vi "Write Caller Enqueuer.vi"(8 "error in (no error)":errorcluster, 10 "Actor Framework:Message Enqueuer":refnum<class "Message Enqueuer.lvclass">, 11 "Async Message in":refnum<class "Async Message.lvclass">) -> (0 "error out":errorcluster, 3 "Async Message out":refnum<class "Async Message.lvclass">)   [LabVIEW 2021, in "Async Methods Actor.lvlib" / "Async Message.lvclass"]
doc: "Sets the caller equeueur to which notify the completion of the Async Method by means of the concreate subclass of the \"Completion Notification Msg.lvclass\" (specified by the \"Completion Notification Msg\" property). The caller will receive the completed Async Message allowing the access by means of it property to its GUID and FQN as well as the remaining number of \"Call and Collect\" Async Messages of the same type. To enable the callee Async Methods Acor to notify completion both this property and the \"Completion Notification Msg\" must be properly set."
uses:
  Async Message.lvclass
  <vilib>/ActorFramework/Message Enqueuer/Message Enqueuer.lvclass
  Async Message.lvclass/Async Message.ctl
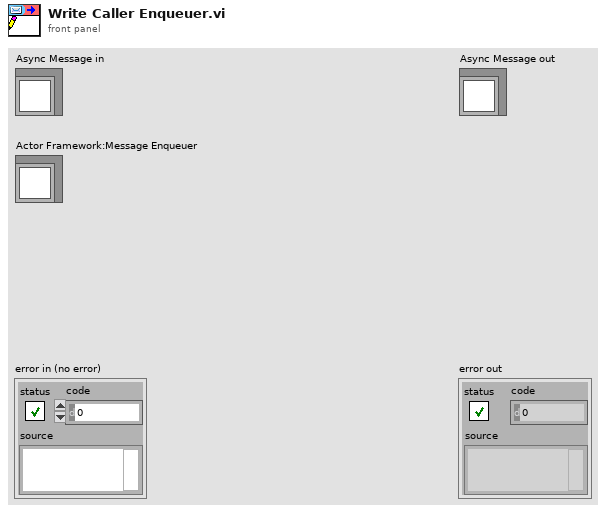
[diagram p1: front panel]
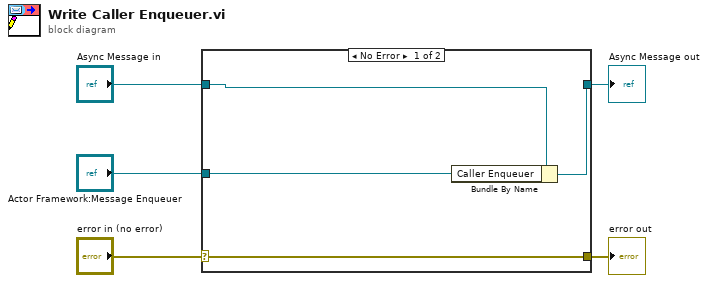
[diagram p0: block diagram]
diagram:
  n1 = case shown="No Error" "error in (no error)" {
    selector: "error in (no error)" -> [w9 w10]
    tunnel: [w9 w10] -> w4
    tunnel: [w8 w11] -> w2
    tunnel: "Async Message in" -> [w6 w11]
    tunnel: "Actor Framework:Message Enqueuer" -> [w7 _]
    frame No Error {
      n2 = Bundle By Name(cluster=w6, "Caller Enqueuer"=w7) -> (w8:refnum<class "Async Message.lvclass">)
    }
    frame Error {
    }
  }
  "error out" <- w4
  "Async Message out" <- w2
